vi "Get param from PGserver.vi"(6 "conninfo":T1={"host"="localhost", "port"="5432", "client_encoding"="WIN1251", "dbname"="data", "user"="postgres", "password"=""}, 8 "error in (no error)":errorcluster, 9 "ParamColumns":string[](array[string])=["value", "value_range_min", "value_range_max", "d", "fname", "value_units", "fcode", "fcodef", "fcode_full"], 10 "ParamTable":string="par_3", 11 "Parameters":string[](array[string])) -> (0 "error out":errorcluster, 2 "Names table":string[][](array[string]), 3 "Parameters table":dbl[][](array[numeric]))   [LabVIEW 2019, in "Inputs.lvlib"]
uses:
  Inputs.lvlib
  Database/ctl/Coninfo.ctl
  Ctl/ParamColumns.ctl
  Database/PostgreSQL2LabVIEW/libpqlv/src/PQfinish.vi
  Database/PostgreSQL2LabVIEW/libpqlv/src/PQconnectdb.vi
  Database/PostgreSQL2LabVIEW/libpqlv/src/PQerrorMessage.vi
  Database/PostgreSQL2LabVIEW/libpqlv/src/PQstatus.vi
  <vilib>/dlg_ctls.llb/Space Constant.vi
  Database/Progress.vi
  Database/PostgreSQL.lvlib
  Database/PostgreSQL2LabVIEW/libpqUtility/libpqutility.lvlib
  Database/PostgreSQL2LabVIEW/libpqUtility64/libpqutility64.lvlib
panel:
  out "PQStatus":T2(ring)
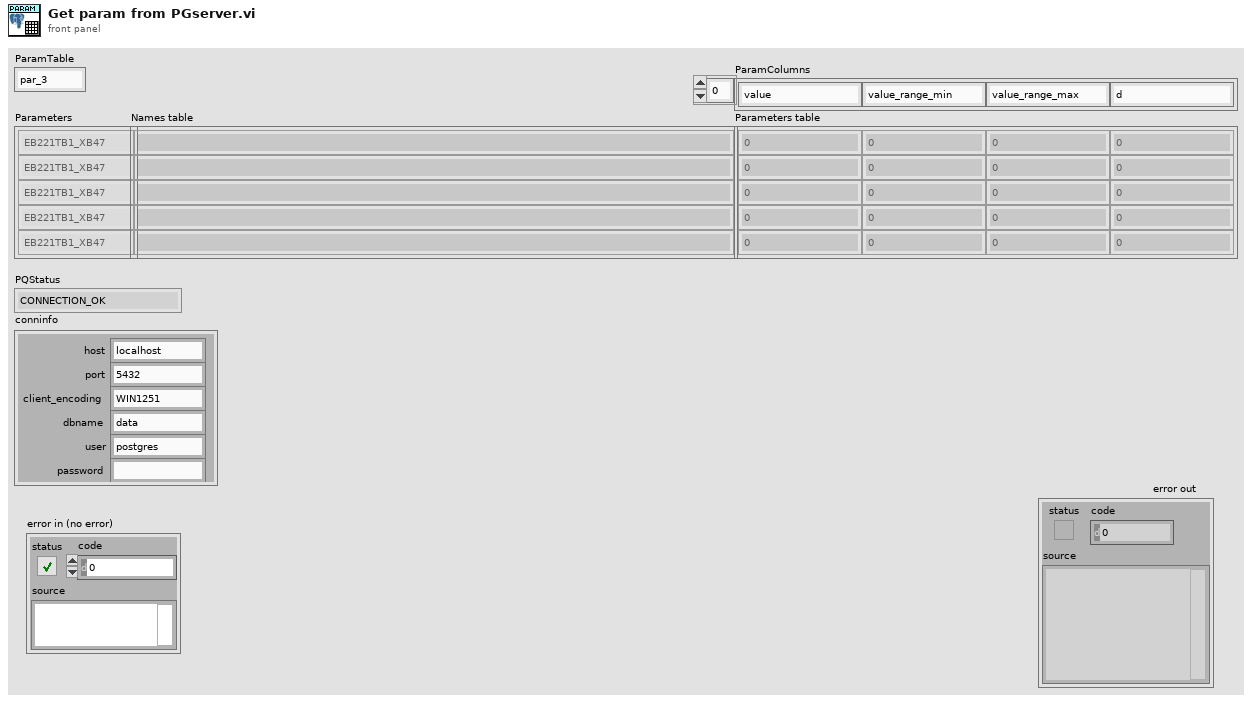
[diagram p1: front panel]
types:
  T1 = typedef "PostgreSQL.lvlib/Coninfo.ctl" = cluster{"host":string, "port":string, "client_encoding":string, "dbname":string, "user":string, "password":string}
  T2 = enum32{"CONNECTION_OK", "CONNECTION_BAD", "CONNECTION_STARTED", "CONNECTION_MADE", "CONNECTION_AWAITING_RESPONSE", "CONNECTION_AUTH_OK", "CONNECTION_SETENV", "CONNECTION_SSL_STARTUP", "CONNECTION_NEEDED"}
  T3 = typedef "Inputs.lvlib/ParamColumns.ctl" = enum16{"value", "value_range_min", "value_range_max", "d", "fname", "value_units", "fcode", "fcodef", "fcode_full"}
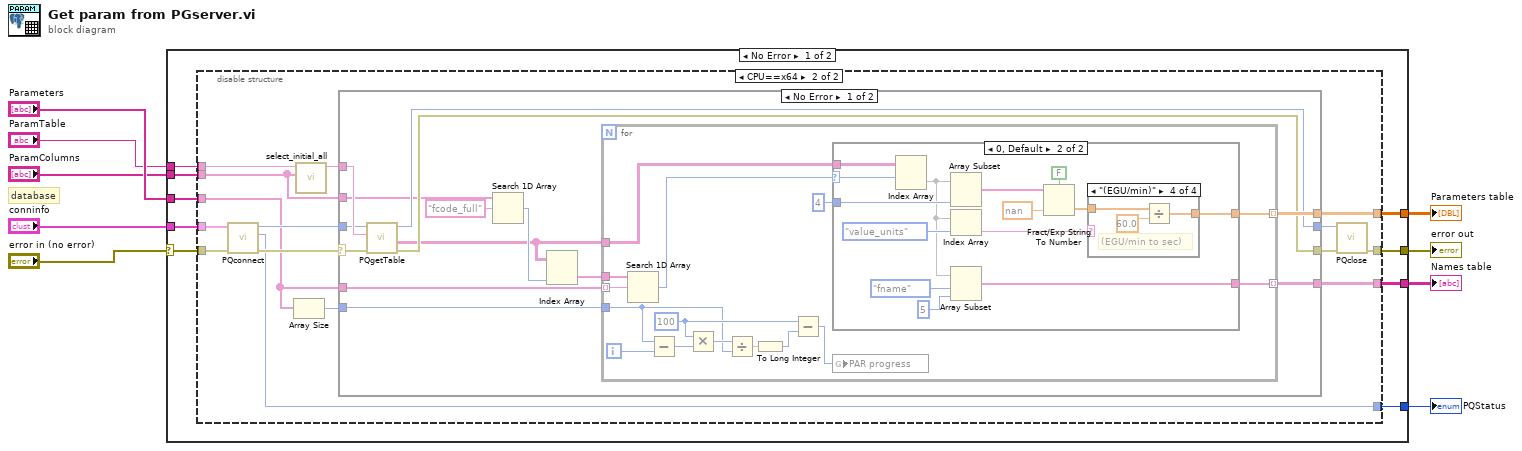
[diagram p0: block diagram]
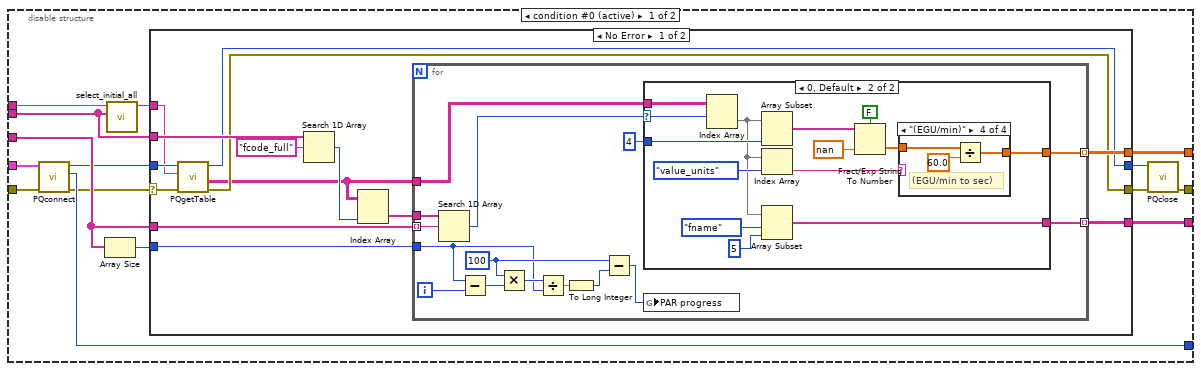
[diagram p2: hidden frame]
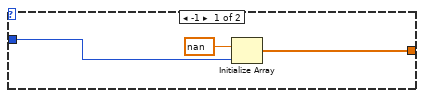
[diagram p3: hidden frame]
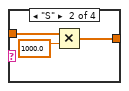
[diagram p5: hidden frame]
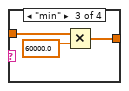
[diagram p6: hidden frame]
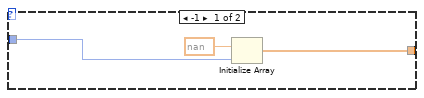
[diagram p8: hidden frame]
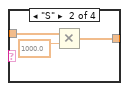
[diagram p10: hidden frame]
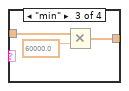
[diagram p11: hidden frame]
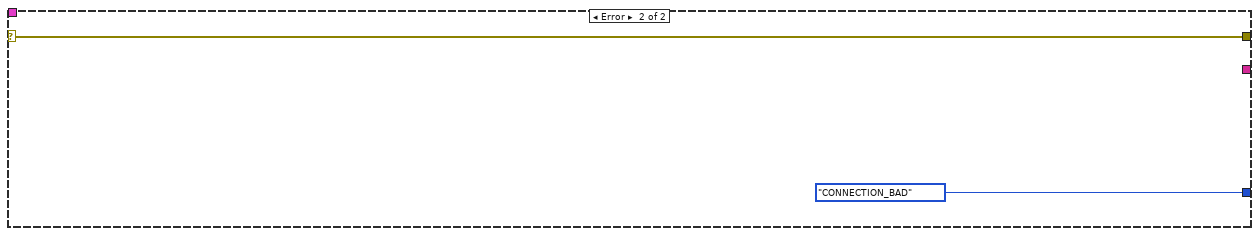
[diagram p13: hidden frame]
diagram:
  # "database"
  n1 = case shown="No Error" "error in (no error)" {
    selector: "error in (no error)" -> [w14 w166]
    tunnel: "Parameters" -> [w18 _]
    tunnel: "ParamTable" -> [w17 _]
    tunnel: "ParamColumns" -> [w16 _]
    tunnel: [w13 _] -> w6
    tunnel: [w12 w166] -> w5
    tunnel: [w11 _] -> w4
    tunnel: "conninfo" -> [w15 _]
    tunnel: [w10 T2."CONNECTION_BAD" ("PQStatus")] -> w1
    frame No Error {
      n2 = disable-structure shown="CPU==x64" {
        disable-tunnel: w18 -> [w29 w101]
        disable-tunnel: w17 -> [w31 w97]
        disable-tunnel: w16 -> [w30 w96]
        disable-tunnel: w15 -> [w25 w100]
        disable-tunnel: w14 -> [w26 w99]
        disable-tunnel: [w27 w95] -> w13
        disable-tunnel: [w20 w94] -> w12
        disable-tunnel: [w28 w93] -> w11
        disable-tunnel: [w23 w92] -> w10
        frame condition #0 (active) {
          n3 = call "PQconnect.vi"("error in (no error)"=w26, "conninfo"=w25) -> ("error out"=w22:errorcluster, "PQStatus"=w23:T2, "conn"=w24:u32)  [unwired: 7 in]
          n4 = Array Size(array=w29) -> (size(s)=w33:i32)
          n5 = call "select_initial_all.vi"("Column table"=w30, "table"=w31) -> ("parameters"=w32:string)  [unwired: 8 in, 1 out]
          n6 = case shown="No Error" w22 {
            selector: w22 -> [w38 w91]
            tunnel: w29 -> [w40 _]
            tunnel: [w47 _] -> w27
            tunnel: [w45 _] -> w28
            tunnel: w33 -> [w46 _]
            tunnel: w24 -> [w39 w90]
            tunnel: w32 -> [w35 _]
            tunnel: [w37 w91] -> w21
            tunnel: [w34 w90] -> w19
            tunnel: w30 -> [w42 _]
            frame No Error {
              n7 = call "PQgetTable.vi"("error in"=w38, "query"=w35, "conn"=w39) -> ("error out"=w37:errorcluster, "Data"=w36:string[][], "conn_out"=w34:u32)  [unwired: 4 in, 2 out]
              n8 = Search 1D Array(1D array=w42, element="fcode_full" ("table")) -> (index of element=w43:i32)  [unwired: 1 in]
              n9 = Index Array(array=w36, index (col)=w43) -> (element=w41:string[])  [unwired: 1 in]
              n10 = for {
                tunnel: [w54] -> w47 mode=indexing
                tunnel: w46 -> [w55]
                tunnel: [w53] -> w45 mode=indexing
                tunnel: w36 -> [w51]
                tunnel: w41 -> [w50]
                tunnel: w40 -> [w49] mode=indexing
                i -> [w56]
                w60 = 100 ("y")
                n11 = Search 1D Array(1D array=w50, element=w49) -> (index of element=w48:i32)  [unwired: 1 in]
                n12 = Subtract(x=w55, y=w56) -> (x-y=w59:i32)
                n13 = Multiply(x=w60, y=w59) -> (x*y=w62:i32)
                n14 = Divide(x=w62, y=w55) -> (x/y=w58:dbl)
                n15 = To Long Integer(number=w58) -> (32bit integer=w57:i32)
                n16 = Subtract(x=w60, y=w57) -> (x-y=w61:i32)
                n17 = case shown="0, Default" w48 {
                  selector: w48 -> [_ w74]
                  tunnel: [w64 w79] -> w54
                  tunnel: 4 -> [w63 w72]
                  tunnel: w51 -> [_ w77]
                  tunnel: [_ w78] -> w53
                  frame -1 {
                    n18 = Initialize Array(nan, w63) -> (w64:dbl[])
                  }
                  frame 0, Default {
                    n19 = Index Array(array=w77, index (row)=w74) -> (element=w69:string[])  [unwired: 1 in]
                    n20 = Array Subset(array=w69, length=w72) -> (w73:string[])  [unwired: 1 in]
                    n21 = Index Array(array=w69, index=ParamColumns."value_units" ("ParamColumns")) -> (element=w71:string)
                    n22 = Array Subset(array=w69, index=ParamColumns."fname" ("ParamColumns"), length=5) -> (w78:string[])
                    n23 = Fract/Exp String To Number(use system decimal point (T)=FALSE, string=w73, default (0 dbl)=nan) -> (number=w66:dbl[])  [unwired: 1 in, 1 out]
                    n24 = case shown="\"(EGU/min)\"" w71 {
                      tunnel: w66 -> [w80 w83 w86 w89]
                      tunnel: [w80 w81 w84 w87] -> w79
                      frame "mS", Default {
                      }
                      frame "S" {
                        n25 = Multiply(x=w83, y=1000.0) -> (x*y=w81:dbl[])
                      }
                      frame "min" {
                        n26 = Multiply(x=w86, y=60000.0) -> (x*y=w84:dbl[])
                      }
                      frame "(EGU/min)" {
                        # "(EGU/min to sec)"
                        n27 = Divide(x=w89, y=60.0) -> (x/y=w87:dbl[])
                      }
                    }
                  }
                }
                n28 = global write "Progress.vi" "PAR progress"(w61) -> ()
              }
            }
            frame Error {
            }
          }
          n29 = call "PQclose.vi"("error in (no error)"=w21, "conn"=w19) -> ("error out"=w20:errorcluster)  [unwired: 9 in]
        }
        frame condition #1 {
          n30 = call "PQconnect.vi"("error in (no error)"=w99, "conninfo"=w100) -> ("error out"=w106:errorcluster, "PQStatus"=w92:T2, "conn"=w103:u64)  [unwired: 7 in]
          n31 = Array Size(array=w101) -> (size(s)=w104:i32)
          n32 = call "select_initial_all.vi"("Column table"=w96, "table"=w97) -> ("parameters"=w98:string)  [unwired: 8 in, 1 out]
          n33 = case shown="No Error" w106 {
            selector: w106 -> [w116 w164]
            tunnel: w101 -> [w107 _]
            tunnel: [w120 _] -> w95
            tunnel: [w118 _] -> w93
            tunnel: w104 -> [w119 _]
            tunnel: w103 -> [w115 w163]
            tunnel: w98 -> [w117 _]
            tunnel: [w114 w164] -> w105
            tunnel: [w113 w163] -> w102
            tunnel: w96 -> [w109 _]
            frame No Error {
              n34 = call "PQgetTable.vi"("error in"=w116, "query"=w117, "conn"=w115) -> ("error out"=w114:errorcluster, "Data"=w110:string[][], "conn_out"=w113:u64)  [unwired: 4 in, 2 out]
              n35 = Search 1D Array(1D array=w109, element="fcode_full" ("table")) -> (index of element=w111:i32)  [unwired: 1 in]
              n36 = Index Array(array=w110, index (col)=w111) -> (element=w108:string[])  [unwired: 1 in]
              n37 = for {
                tunnel: [w127] -> w120 mode=indexing
                tunnel: w119 -> [w128]
                tunnel: [w126] -> w118 mode=indexing
                tunnel: w110 -> [w124]
                tunnel: w108 -> [w123]
                tunnel: w107 -> [w122] mode=indexing
                i -> [w129]
                w133 = 100 ("y")
                n38 = Search 1D Array(1D array=w123, element=w122) -> (index of element=w121:i32)  [unwired: 1 in]
                n39 = Subtract(x=w128, y=w129) -> (x-y=w132:i32)
                n40 = Multiply(x=w133, y=w132) -> (x*y=w135:i32)
                n41 = Divide(x=w135, y=w128) -> (x/y=w131:dbl)
                n42 = To Long Integer(number=w131) -> (32bit integer=w130:i32)
                n43 = Subtract(x=w133, y=w130) -> (x-y=w134:i32)
                n44 = case shown="0, Default" w121 {
                  selector: w121 -> [_ w147]
                  tunnel: [w137 w152] -> w127
                  tunnel: 4 -> [w136 w145]
                  tunnel: w124 -> [_ w150]
                  tunnel: [_ w151] -> w126
                  frame -1 {
                    n45 = Initialize Array(nan, w136) -> (w137:dbl[])
                  }
                  frame 0, Default {
                    n46 = Index Array(array=w150, index (row)=w147) -> (element=w142:string[])  [unwired: 1 in]
                    n47 = Array Subset(array=w142, length=w145) -> (w146:string[])  [unwired: 1 in]
                    n48 = Index Array(array=w142, index=ParamColumns."value_units" ("ParamColumns")) -> (element=w144:string)
                    n49 = Array Subset(array=w142, index=ParamColumns."fname" ("ParamColumns"), length=5) -> (w151:string[])
                    n50 = Fract/Exp String To Number(use system decimal point (T)=FALSE, string=w146, default (0 dbl)=nan) -> (number=w139:dbl[])  [unwired: 1 in, 1 out]
                    n51 = case shown="\"(EGU/min)\"" w144 {
                      tunnel: w139 -> [w153 w156 w159 w162]
                      tunnel: [w153 w154 w157 w160] -> w152
                      frame "mS", Default {
                      }
                      frame "S" {
                        n52 = Multiply(x=w156, y=1000.0) -> (x*y=w154:dbl[])
                      }
                      frame "min" {
                        n53 = Multiply(x=w159, y=60000.0) -> (x*y=w157:dbl[])
                      }
                      frame "(EGU/min)" {
                        # "(EGU/min to sec)"
                        n54 = Divide(x=w162, y=60.0) -> (x/y=w160:dbl[])
                      }
                    }
                  }
                }
                n55 = global write "Progress.vi" "PAR progress"(w134) -> ()
              }
            }
            frame Error {
            }
          }
          n56 = call "PQclose.vi"("error in (no error)"=w105, "conn"=w102) -> ("error out"=w94:errorcluster)  [unwired: 9 in]
        }
      }
    }
    frame Error {
    }
  }
  "error out" <- w5
  "Parameters table" <- w6
  "Names table" <- w4
  "PQStatus" <- w1
